vi "Tag_Value_Entry_PopUp.vi"(6 "Write Type":enum16{"SetRequest", "WriteValue"}(ring), 7 "Namespace":string, 8 "error in (no error)":errorcluster, 9 "Timeout (-1)":i32=-1, 10 "Synchronous (F)":bool, 11 "Tag Name":string) -> (0 "error out":errorcluster, 1 "found":bool, 2 "New Value":variant, 3 "Apply":bool)   [LabVIEW 2018, in "Tag Watchlist.lvlib"]
uses:
  Tag Watchlist.lvlib
  Core/Tag Core.lvclass/Tag Core.ctl
  Tag/Tag.lvclass/Tag.ctl
  3d21ca5b-4206-44a6-9f4a-353a7ad2adf7.vi
  c034b9bb-27a6-4754-8b85-6793f2d11a0f.vi
  Tag/Read Type.vi
  Tag/Read Value.vi
  Tag/Write SetRequest.vi
  Tag/Write Value with Timestamp.vi
  Core/Get Tag LUT.vi
  <vilib>/Utility/error.llb/Error Cluster From Error Code.vi
  Tag/Tag.lvclass
  Core/Tag Core.lvclass
panel:
  # "!!! Write Value is for debugging purposes only !!"
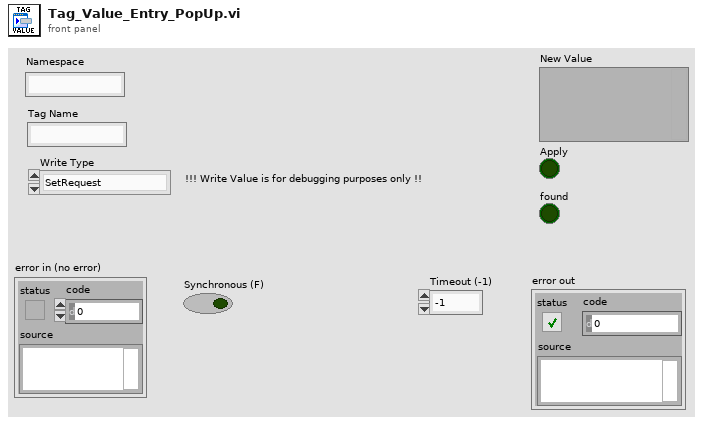
[diagram p1: front panel]
types:
  T1 = typedef "NI_Data Type.lvlib/Data Type.ctl" = enum8{"Invalid Type", "Void", "I8", "I16", "I32", "I64", "U8", "U16", "U32", "U64", "Single Float", "Double Float", "Extended Float", "Single Complex", "Double Complex", "Extended Complex", "Enum U8", "Enum U16", "Enum U32", "Enum U64", "Single Float With Unit", "Double Float With Unit", "Extended Float With Unit", "Single Complex with Unit", "Double Complex with Unit", "Extended Complex with Unit", "Boolean", "String", "Path", "Picture", "Tag", "Array", "Cluster", "Variant", "LV Variant", "Waveform", "Timestamp", "Digital Waveform", "Digital Data", "ExpressData", "Refnum", "External Data", "VI", "Poly VI", "LabVIEW Class Instance", "Fixed Point"}
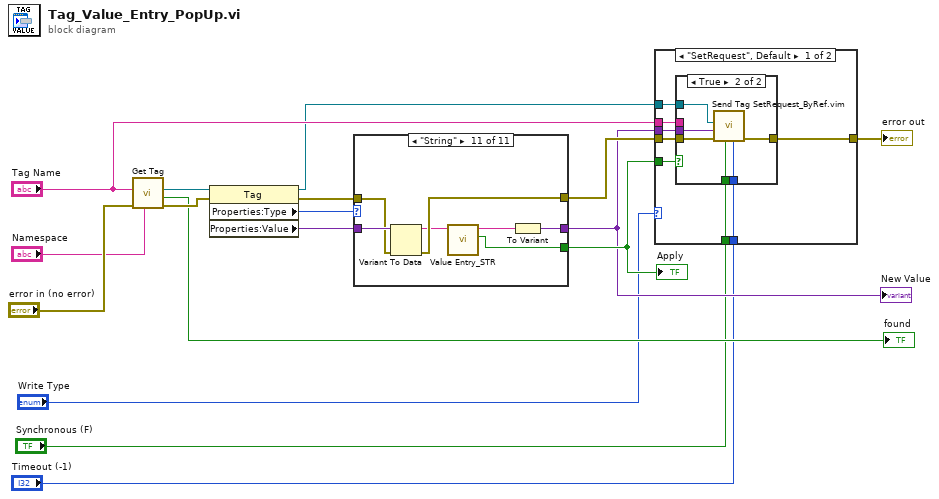
[diagram p0: block diagram]
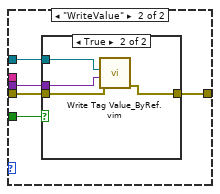
[diagram p3: hidden frame]
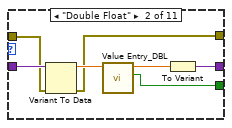
[diagram p6: hidden frame]
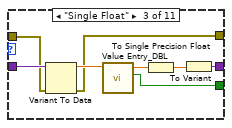
[diagram p7: hidden frame]
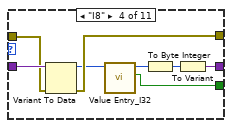
[diagram p8: hidden frame]
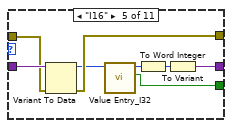
[diagram p9: hidden frame]
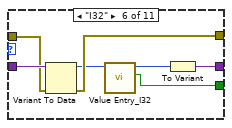
[diagram p10: hidden frame]
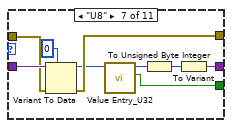
[diagram p11: hidden frame]
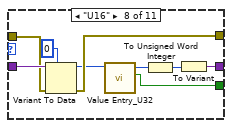
[diagram p12: hidden frame]
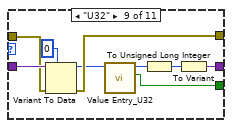
[diagram p13: hidden frame]
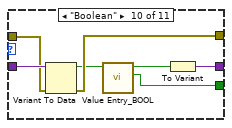
[diagram p14: hidden frame]
diagram:
  n1 = call "Get Tag.vi"("Namespace"="Namespace", "error in (no error)"="error in (no error)", "Name"="Tag Name") -> ("error out"=w7:errorcluster, "found"=→"found":bool, "Tag Ref out"=w17:refnum<data-value>)  [unwired: 6 in]
  n2 = property class="Tag"(reference=w17, error in=w7) -> (reference out=w4:refnum<data-value>, error out=w13:errorcluster, "Properties:Type"=w16:T1, "Properties:Value"=w15:variant)
  n3 = case shown="\"String\"" w16 {
    tunnel: w15 -> [w18 w26 w34 w42 w50 w57 w66 w75 w84 w91 w98]
    tunnel: w13 -> [w19 w24 w32 w41 w49 w56 w65 w74 w83 w90 w97]
    tunnel: [w19 w23 w31 w40 w48 w55 w64 w73 w82 w89 w96] -> w12
    tunnel: [_ w21 w30 w37 w45 w52 w61 w70 w79 w85 w92] -> w11
    tunnel: [w18 w20 w29 w39 w47 w54 w63 w72 w81 w88 w95] -> w9
    frame "Variant", Default {
    }
    frame "Double Float" {
      n4 = Variant To Data(error in=w24, Variant=w26) -> (data=w25:dbl, error out=w23:errorcluster)  [unwired: 1 in]
      n5 = call "Value Entry_DBL.vi"("Value In"=w25) -> ("Apply"=w21:bool, "Value Out"=w22:dbl)  [unwired: 9 in]
      n6 = To Variant(anything=w22) -> (Variant=w20:variant)
    }
    frame "Single Float" {
      n7 = Variant To Data(error in=w32, Variant=w34) -> (data=w33:dbl, error out=w31:errorcluster)  [unwired: 1 in]
      n8 = call "Value Entry_DBL.vi"("Value In"=w33) -> ("Apply"=w30:bool, "Value Out"=w28:dbl)  [unwired: 9 in]
      n9 = To Single Precision Float(number=w28) -> (single precision float=w27:sgl)
      n10 = To Variant(anything=w27) -> (Variant=w29:variant)
    }
    frame "I8" {
      n11 = Variant To Data(error in=w41, Variant=w42) -> (data=w38:i32, error out=w40:errorcluster)  [unwired: 1 in]
      n12 = call "Value Entry_I32.vi"("Value In"=w38) -> ("Apply"=w37:bool, "Value Out"=w36:i32)  [unwired: 9 in]
      n13 = To Byte Integer(number=w36) -> (8bit integer=w35:i8)
      n14 = To Variant(anything=w35) -> (Variant=w39:variant)
    }
    frame "I16" {
      n15 = Variant To Data(error in=w49, Variant=w50) -> (data=w46:i32, error out=w48:errorcluster)  [unwired: 1 in]
      n16 = call "Value Entry_I32.vi"("Value In"=w46) -> ("Apply"=w45:bool, "Value Out"=w44:i32)  [unwired: 9 in]
      n17 = To Word Integer(number=w44) -> (16bit integer=w43:i16)
      n18 = To Variant(anything=w43) -> (Variant=w47:variant)
    }
    frame "I32" {
      n19 = Variant To Data(error in=w56, Variant=w57) -> (data=w53:i32, error out=w55:errorcluster)  [unwired: 1 in]
      n20 = call "Value Entry_I32.vi"("Value In"=w53) -> ("Apply"=w52:bool, "Value Out"=w51:i32)  [unwired: 9 in]
      n21 = To Variant(anything=w51) -> (Variant=w54:variant)
    }
    frame "U8" {
      n22 = Variant To Data(error in=w65, type=u32 0, Variant=w66) -> (data=w62:u32, error out=w64:errorcluster)
      n23 = call "Value Entry_U32.vi"("Value In"=w62) -> ("Apply"=w61:bool, "Value Out"=w58:u32)  [unwired: 9 in]
      n24 = To Unsigned Byte Integer(number=w58) -> (unsigned 8bit integer=w59:u8)
      n25 = To Variant(anything=w59) -> (Variant=w63:variant)
    }
    frame "U16" {
      n26 = Variant To Data(error in=w74, type=u32 0, Variant=w75) -> (data=w71:u32, error out=w73:errorcluster)
      n27 = call "Value Entry_U32.vi"("Value In"=w71) -> ("Apply"=w70:bool, "Value Out"=w68:u32)  [unwired: 9 in]
      n28 = To Unsigned Word Integer(number=w68) -> (unsigned 16bit integer=w67:u16)
      n29 = To Variant(anything=w67) -> (Variant=w72:variant)
    }
    frame "U32" {
      n30 = Variant To Data(error in=w83, type=u32 0, Variant=w84) -> (data=w80:u32, error out=w82:errorcluster)
      n31 = call "Value Entry_U32.vi"("Value In"=w80) -> ("Apply"=w79:bool, "Value Out"=w77:u32)  [unwired: 9 in]
      n32 = To Unsigned Long Integer(number=w77) -> (unsigned 32bit integer=w76:u32)
      n33 = To Variant(anything=w76) -> (Variant=w81:variant)
    }
    frame "Boolean" {
      n34 = Variant To Data(error in=w90, Variant=w91) -> (data=w86:bool, error out=w89:errorcluster)  [unwired: 1 in]
      n35 = call "Value Entry_BOOL.vi"("Value In"=w86) -> ("Apply"=w85:bool, "Value Out"=w87:bool)  [unwired: 9 in]
      n36 = To Variant(anything=w87) -> (Variant=w88:variant)
    }
    frame "String" {
      n37 = Variant To Data(error in=w97, Variant=w98) -> (data=w93:string, error out=w96:errorcluster)  [unwired: 1 in]
      n38 = call "Value Entry_STR.vi"("Value In"=w93) -> ("Apply"=w92:bool, "Value Out"=w94:string)  [unwired: 9 in]
      n39 = To Variant(anything=w94) -> (Variant=w95:variant)
    }
  }
  "New Value" <- w9
  "Apply" <- w11
  n40 = case shown="\"SetRequest\", Default" "Write Type" {
    tunnel: "Tag Name" -> [w106 _]
    tunnel: w12 -> [w105 w117]
    tunnel: w11 -> [w104 w118]
    tunnel: [w103 w114] -> w10
    tunnel: w9 -> [w102 w116]
    tunnel: w4 -> [w99 w115]
    tunnel: "Synchronous (F)" -> [w101 _]
    tunnel: "Timeout (-1)" -> [w100 _]
    frame "SetRequest", Default {
      n41 = case shown="True" w104 {
        tunnel: w106 -> [_ _]
        tunnel: w105 -> [w107 w113]
        tunnel: [w107 w112] -> w103
        tunnel: w102 -> [_ w111]
        tunnel: w101 -> [_ w110]
        tunnel: w100 -> [_ w109]
        tunnel: w99 -> [_ w108]
        frame False {
        }
        frame True {
          n42 = call "Send Tag SetRequest_ByRef.vim"("Timeout (-1)"=w109, "Synchronous (F)"=w110, "error in (no error)"=w113, "Value"=w111, "Tag Ref in"=w108) -> ("error out"=w112:errorcluster)  [unwired: 4 in, 2 out]
        }
      }
    }
    frame "WriteValue" {
      n43 = case shown="True" w118 {
        tunnel: w117 -> [w119 w121]
        tunnel: w116 -> [_ w122]
        tunnel: w115 -> [_ w123]
        tunnel: [w119 w120] -> w114
        frame False {
        }
        frame True {
          n44 = call "Write Tag Value_ByRef.vim"("error in (no error)"=w121, "Value"=w122, "Tag Ref in"=w123) -> ("error out"=w120:errorcluster)  [unwired: 7 in, 1 out]
        }
      }
    }
  }
  "error out" <- w10
